vi "zaber_raw_command.vi"(8 "error in (no error)":errorcluster, 9 "Device and Axis":string, 10 "Command":string, 11 "VISA Refnum in":refnum<visa-resource-name>) -> (0 "error out":errorcluster, 1 "First Response Device Number":string, 2 "Response Bundle Array":T1(array[cluster]), 3 "VISA resource name out":refnum<visa-resource-name>, 4 "Response String Array":string[](array[string]), 5 "First Response Data Value":string)   [LabVIEW 2020, in "ZaberASeries.lvclass"]
uses:
  ZaberASeries.lvclass
  Zaber A Series.lvlib
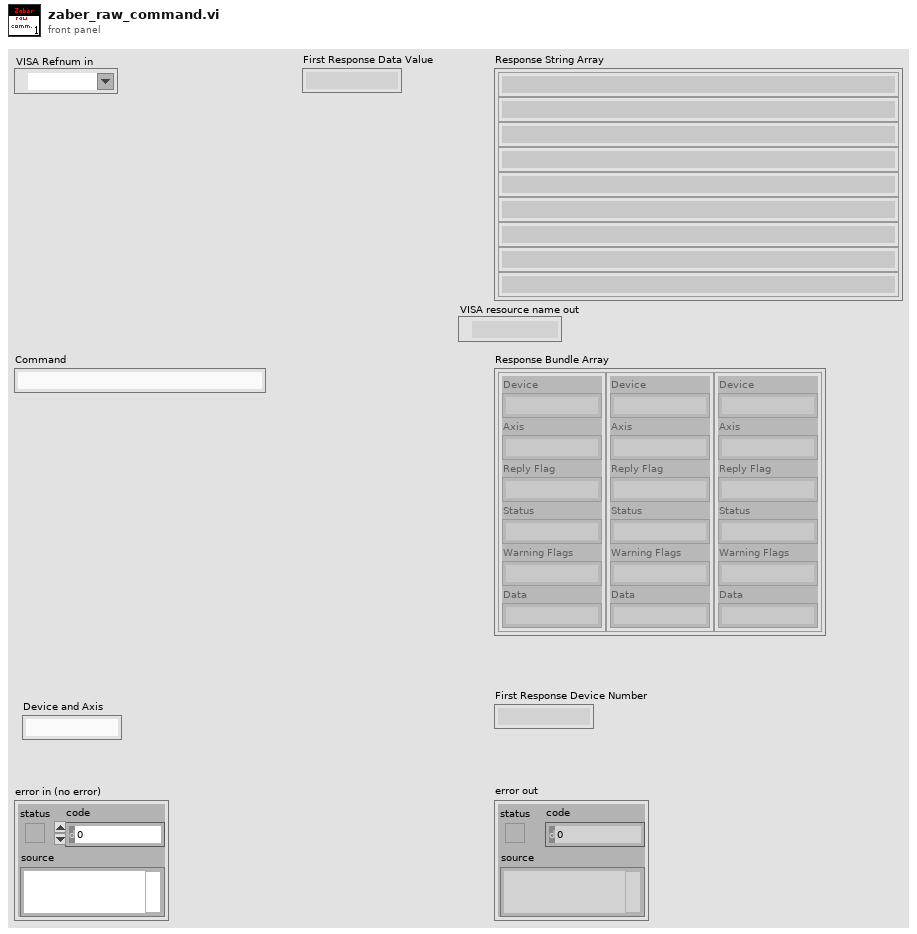
[diagram p1: front panel]
types:
  T1 = cluster{"Device":string, "Axis":string, "Reply Flag":string, "Status":string, "Warning Flags":string, "Data":string}[]
  T2 = cluster{"Device":string, "Axis":string, "Reply Flag":string, "Status":string, "Warning Flags":string, "Data":string}
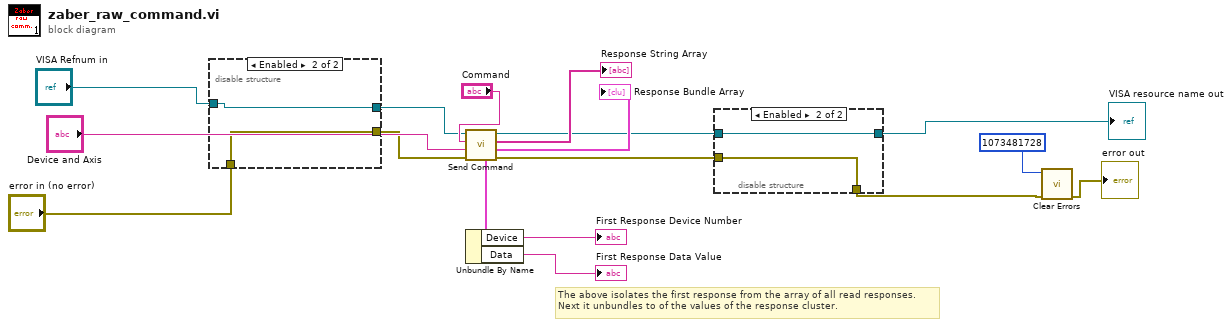
[diagram p0: block diagram]
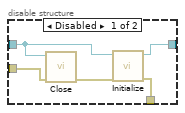
[diagram p2: hidden frame]
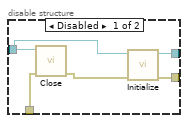
[diagram p3: hidden frame]
diagram:
  # "The above isolates the first response from the array of all read responses.\nNext it unbundles to of the values of the response cluster."
  n1 = disable-structure shown="Enabled" {
    disable-tunnel: "error in (no error)" -> [w22 w23]
    disable-tunnel: "VISA Refnum in" -> [w20 w24]
    disable-tunnel: [w19 w24] -> w6
    disable-tunnel: [w18 w23] -> w5
    frame Disabled {
      n2 = call "Close.vi"("error in (no error)"=w22, "VISA resource name"=w20) -> ("error out"=w21:errorcluster)  [unwired: 9 in]
      n3 = call "Initialize.vi"("error in (no error)"=w21, "VISA resource name"=w20) -> ("error out"=w18:errorcluster, "VISA resource name out"=w19:refnum<visa-resource-name>)  [unwired: 8 in]
    }
    frame Enabled {
    }
  }
  n4 = call "Send Command.vi"("error in (no error)"=w5, "Device and Axis"="Device and Axis", "Command"="Command", "VISA resource name"=w6) -> ("error out"=w2:errorcluster, "Response Bundle Array"=→"Response Bundle Array":T1, "Response String Array"=→"Response String Array":string[], "VISA resource name out"=w4:refnum<visa-resource-name>, "First Response Bundle"=w15:T2)  [unwired: 2 in, 1 out]
  n5 = Unbundle By Name(w15) -> ("Device"=→"First Response Device Number":string, "Data"=→"First Response Data Value":string)
  n6 = disable-structure shown="Enabled" {
    disable-tunnel: w4 -> [w29 w31]
    disable-tunnel: [w28 w31] -> w3
    disable-tunnel: w2 -> [w26 w30]
    disable-tunnel: [w25 w30] -> w1
    frame Disabled {
      n7 = call "Close.vi"("error in (no error)"=w26, "VISA resource name"=w29) -> ("error out"=w27:errorcluster)  [unwired: 9 in]
      n8 = call "Initialize.vi"("error in (no error)"=w27, "VISA resource name"=w29) -> ("error out"=w25:errorcluster, "VISA resource name out"=w28:refnum<visa-resource-name>)  [unwired: 8 in]
    }
    frame Enabled {
    }
  }
  "VISA resource name out" <- w3
  n9 = call <vilib>:"Clear Errors.vi"("error in (no error)"=w1, "specific error code to clear (0: all)"=1073481728) -> ("error out"=→"error out":errorcluster)  [unwired: 4 in, 1 out]
